vi "SVT Zoom Power Spectral Density.vi"   [LabVIEW 2017]
doc: "Computes the zoom power spectral density based on <B>scaled signal [EU]</B> and <B>zoom settings</B>. Data is accumulated each time this VI is called. However, it returns a new spectrum only when sufficient data has been accumulated. Indicators and subsequent processing should only be called when <B>new spectrum available</B> is TRUE. You can use this polymorphic VI to analyze signals from a single channel or from N channels. The data type you wire to the <B>scaled signal [EU]</B> input determines the polymorphic instance to use."
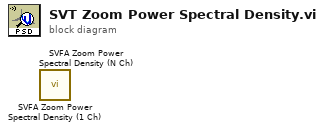
[diagram p0: block diagram]
diagram:
  n1 = call <vilib>:"SVFA Zoom Power Spectral Density (1 Ch).vi"() -> ()  [unwired: 13 in, 7 out]
  n2 = call <vilib>:"SVFA Zoom Power Spectral Density (N Ch).vi"() -> ()  [unwired: 13 in, 7 out]
